vi "Get Next State.vi"(11 "Main Array":T2={"FIFO Array"=[{"Auto States"=enum."Initilize", "Dist"=4.3, "Radians"=0.0, "MaxSpeed (ft/s)"=1.2, "TimeOut (s)"=10.0, "CMD"="", "ArmSetpoints"=enum."ShoulderRest"}], "Dist (ft)"=0.0, "MaxSpeed (ft/s)"=0.0, "TimeOut (s)"=99.0, "Timer Value"=0, "DriveStraightDistance"=[], "ModuleTravelPosition"=[0.0, 0.0, 0.0, 0.0], "First Time"=FALSE, "Current Step"={"Auto States"=enum."Unknown", "Dist"=4.3, "Radians"=0.0, "MaxSpeed (ft/s)"=1.2, "TimeOut (s)"=10.0, "CMD"="", "ArmSetpoints"=enum."ShoulderRest"}}) -> (1 "Next State":T1, 3 "Main Array out":T2={"FIFO Array"=[{"Auto States"=enum."Initilize", "Dist"=4.3, "Radians"=0.0, "MaxSpeed (ft/s)"=1.2, "TimeOut (s)"=10.0, "CMD"="", "ArmSetpoints"=enum."ShoulderRest"}], "Dist (ft)"=0.0, "MaxSpeed (ft/s)"=0.0, "TimeOut (s)"=99.0, "Timer Value"=0, "DriveStraightDistance"=[], "ModuleTravelPosition"=[0.0, 0.0, 0.0, 0.0], "First Time"=FALSE, "Current Step"={"Auto States"=enum."Unknown", "Dist"=4.3, "Radians"=0.0, "MaxSpeed (ft/s)"=1.2, "TimeOut (s)"=10.0, "CMD"="", "ArmSetpoints"=enum."ShoulderRest"}})   [LabVIEW 2023]
uses:
  Auot FIFO.ctl
  Auton Main Array.ctl
  FIFO Array.ctl
  Auot States.ctl
  Shoulder/ShoulderGetSetpointEnum.ctl
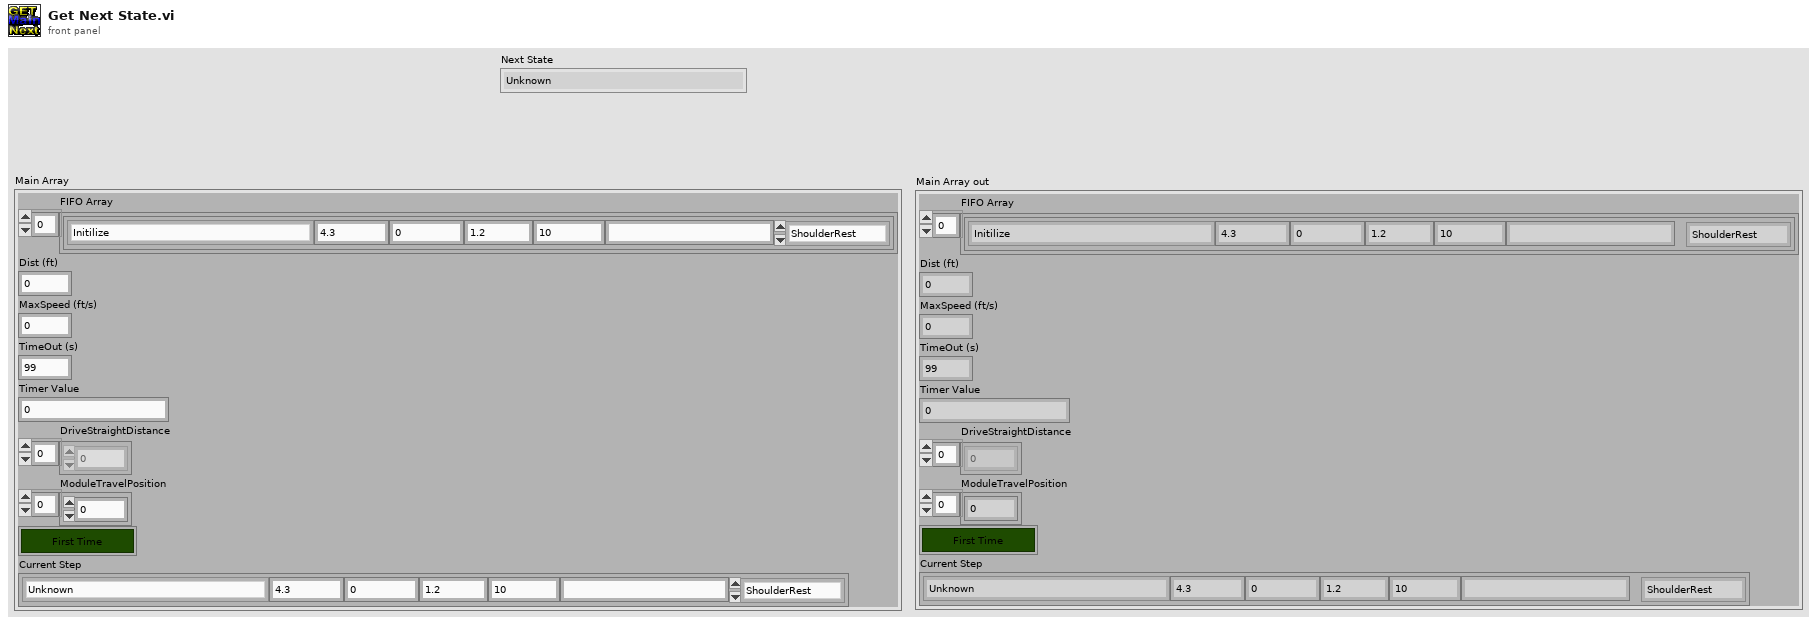
[diagram p1: front panel]
types:
  T1 = typedef "Auot States.ctl" = enum16{"Unknown", "Initilize", "Intake", "Move Arm", "Drive Straight", "Drive Trajorctory", "Drive Turn", "Send Bool CMD", "Set Target", "Shoot", "Wait", "Exit"}
  T2 = typedef "Auton Main Array.ctl" = cluster{"FIFO Array":T3, "Dist (ft)":dbl, "MaxSpeed (ft/s)":dbl, "TimeOut (s)":dbl, "Timer Value":u32, "DriveStraightDistance":dbl[], "ModuleTravelPosition":dbl[], "First Time":bool, "Current Step":T4}
  T3 = typedef "FIFO Array.ctl" = T4[]
  T4 = typedef "Auot FIFO.ctl" = cluster{"Auto States":T1, "Dist":dbl, "Radians":dbl, "MaxSpeed (ft/s)":dbl, "TimeOut (s)":dbl, "CMD":string, "ArmSetpoints":T5}
  T5 = typedef "ShoulderGetSetpointEnum.ctl" = enum16{"Select", "ShoulderRest", "ShoulderSpeaker", "ShoulderAmp"}
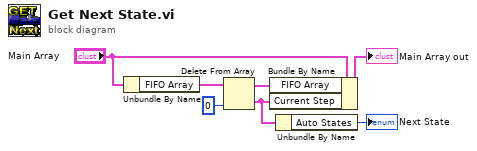
[diagram p0: block diagram]
diagram:
  n1 = Unbundle By Name("Main Array") -> ("FIFO Array"=w7:T3)
  n2 = Delete From Array(array=w7, index=0) -> (deleted portion=w1:T4, array with subset deleted=w4:T3)  [unwired: 1 in]
  n3 = Bundle By Name(cluster="Main Array", "FIFO Array"=w4, "Current Step"=w1) -> (→"Main Array out":T2)
  n4 = Unbundle By Name(w1) -> ("Auto States"=→"Next State":T1)
